vi "comet_thermo_get_serial_MODBUS.vi"(8 "error in":errorcluster, 11 "TCP ref in":refnum<k5>) -> (0 "error out":errorcluster, 1 "ID string (virtual)":string, 2 "serial string":string, 3 "TCP ref out":refnum<k5>)   [LabVIEW 2013]
uses:
  NI Modbus.llb/MB Modbus Command.ctl
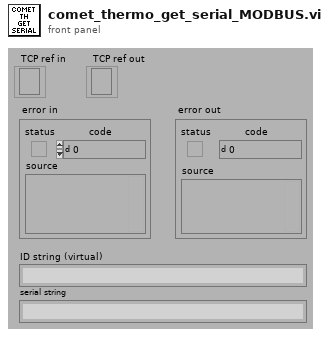
[diagram p1: front panel]
types:
  T1 = typedef "MB Modbus Command.ctl" = cluster{"Function Code":u8, "Starting Address":u16, "Quantity":u16, "Data":u16[], "Discrete":bool[]}
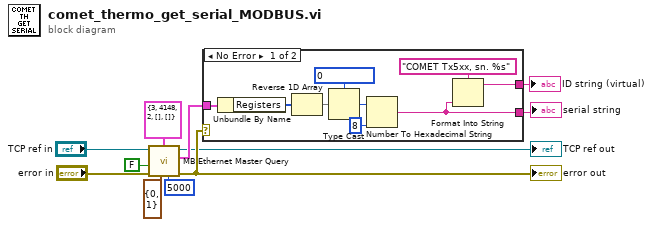
[diagram p0: block diagram]
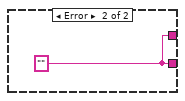
[diagram p2: hidden frame]
diagram:
  n1 = call "MB Ethernet Master Query.vi"("Timeout"=5000, "MBAP Header"=cluster{"Transaction ID":u16, "Unit ID":u8} {"Transaction ID"=0, "Unit ID"=1}, "error in (no error)"="error in", "Use MODBUS Data Unit?"=FALSE, "Modbus Command"=T1 {"Function Code"=3, "Starting Address"=4148, "Quantity"=2, "Data"=[], "Discrete"=[]}, "TCP Connection Refnum in"="TCP ref in") -> ("error out"=w4:errorcluster, "Registers"=w7:cluster{"Registers":u16[], "Discrete":bool[]}, "TCP Connection Refnum (dup)"=→"TCP ref out":refnum<k5>)  [unwired: 1 in, 2 out]
  "error out" <- w4
  n2 = case shown="No Error" w4 {
    tunnel: w7 -> [w20 _]
    tunnel: [w13 w21] -> w5
    tunnel: [w12 w21] -> w1
    frame No Error {
      n3 = Unbundle By Name(w20) -> ("Registers"=w19:u16[])
      n4 = Reverse 1D Array(array=w19) -> (reversed array=w15:u16[])
      n5 = Type Cast(type=u32 0, x=w15) -> (*(type *) &x=w17:u32)
      n6 = Number To Hexadecimal String(1:i16 8 ("width (-)"), 2:w17) -> (0:w13:string)
      n7 = Format Into String(format string="COMET Tx5xx, sn. %s", w13) -> (resulting string=w12:string)  [unwired: 2 in, 1 out]
    }
    frame Error {
      w21 = ""
    }
  }
  "serial string" <- w5
  "ID string (virtual)" <- w1
